vi "ReadNortekFile.vi"(4 "error in":errorcluster, 7 "FichierNortek":path) -> (0 "error out":errorcluster, 2 "Nortek WaveForms":waveform(dbl)[](graph))   [LabVIEW 2017]
uses:
  <vilib>/gmath/NI_Gmath.lvlib
panel:
  out "text":string
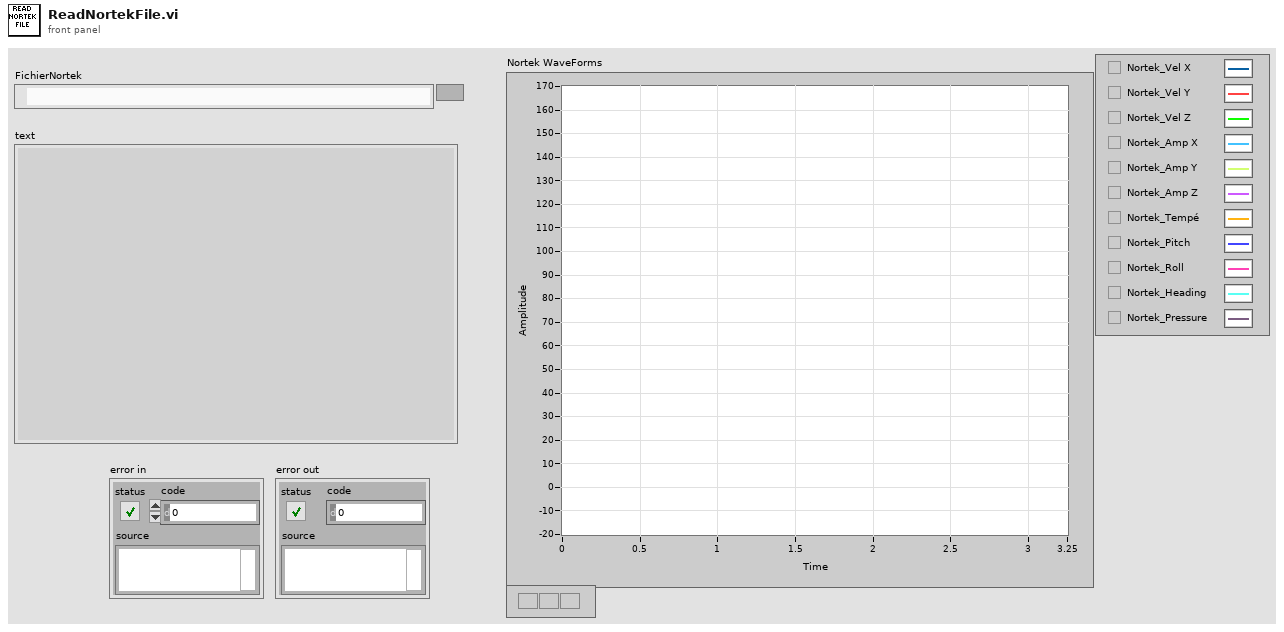
[diagram p1: front panel]
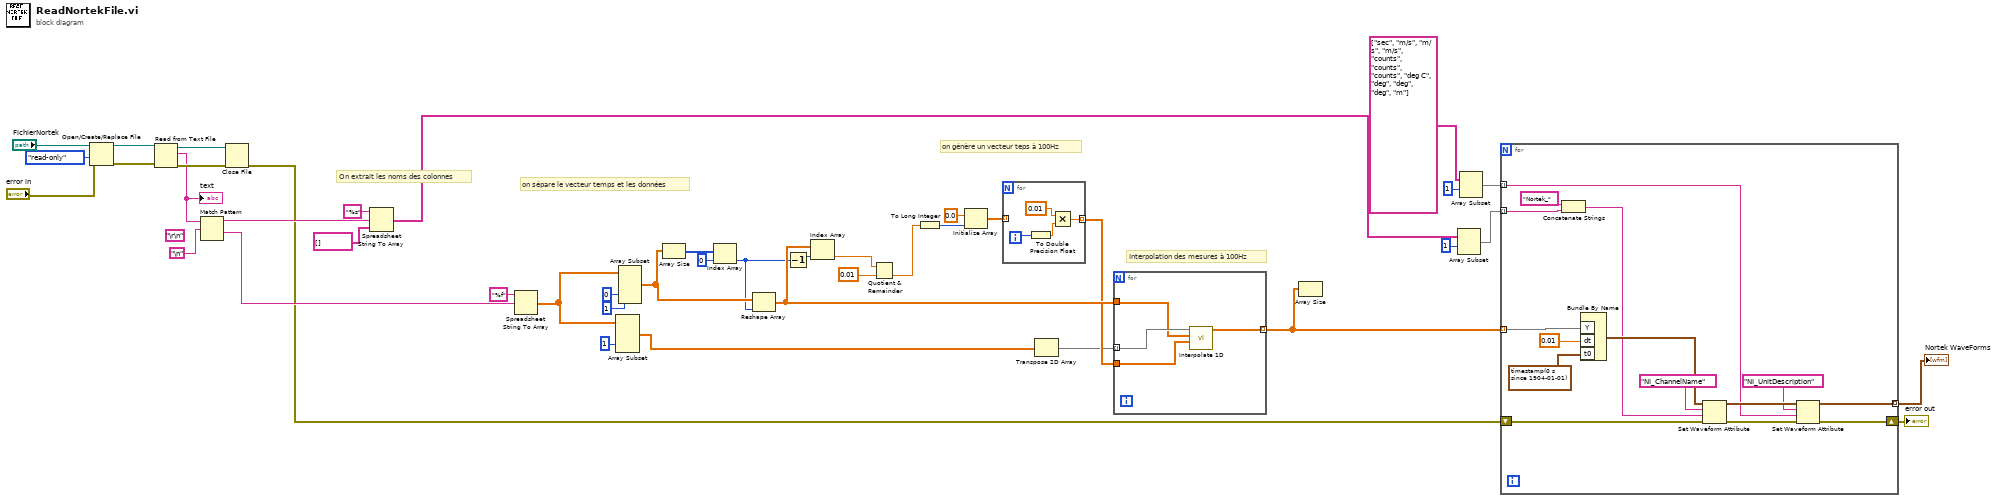
[diagram p0: block diagram]
diagram:
  (unwired) "\r\n"
  # "Interpolation des mesures à 100Hz"
  # "on génère un vecteur teps à 100Hz"
  # "on sépare le vecteur temps et les données"
  # "On extrait les noms des colonnes"
  n1 = Open/Create/Replace File(file path (use dialog)="FichierNortek", error in="error in", access (0:read/write)=enum16{"read/write", "read-only", "write-only"}."read-only") -> (refnum out=w41:refnum<file>, error out=w43:errorcluster)  [unwired: 3 in, 1 out]
  n2 = Read from Text File(file (use dialog)=w41, error in=w43) -> (refnum out=w40:refnum<file>, text=w36:string, error out=w42:errorcluster)  [unwired: 2 in, 1 out]
  "text" <- w36
  n3 = Match Pattern(string=w36, regular expression="\n") -> (before substring=w34:string, after substring=w31:string)  [unwired: 1 in, 2 out]
  n4 = Close File(refnum=w40, error in=w42) -> (error out=w9:errorcluster)  [unwired: 1 out]
  n5 = Spreadsheet String To Array(format string="%s", spreadsheet string=w34, array type (2D Dbl)=string[] []) -> (array=w2:string[])  [unwired: 1 in]
  n6 = Spreadsheet String To Array(format string="%f", spreadsheet string=w31) -> (array=w26:dbl[][])  [unwired: 2 in]
  n7 = Array Subset(array=w26, index (col)=1 ("index")) -> (w25:dbl[][])  [unwired: 3 in]
  n8 = Array Subset(array=w26, index (col)=0 ("index"), length (col)=1 ("length")) -> (w24:dbl[][])  [unwired: 2 in]
  n9 = Array Size(array=w24) -> (size(s)=w23:i32[])
  n10 = Index Array(array=w23, index=0) -> (element=w20:i32)
  n11 = Reshape Array(w24, w20) -> (w21:dbl[])
  n12 = Decrement(x=w20) -> (x-1=w19:i32)
  n13 = Index Array(array=w21, index=w19) -> (element=w18:dbl)
  n14 = Quotient & Remainder(x=w18, y=0.01) -> (floor(x/y)=w16:dbl)  [unwired: 1 out]
  n15 = To Long Integer(number=w16) -> (32bit integer=w15:i32)
  n16 = Initialize Array(0.0 ("element"), w15) -> (w13:dbl[])
  n17 = for {
    tunnel: w13 -> [_] mode=indexing
    tunnel: [w45] -> w12 mode=indexing
    i -> [w46]
    n18 = To Double Precision Float(number=w46) -> (double precision float=w44:dbl)
    n19 = Multiply(x=0.01 ("y"), y=w44) -> (x*y=w45:dbl)
  }
  n20 = Transpose 2D Array(2D array=w25) -> (transposed array=w11:dbl[][])
  n21 = for {
    tunnel: w11 -> [w51] mode=indexing
    tunnel: w21 -> [w50]
    tunnel: w12 -> [w49]
    tunnel: [w48] -> w10 mode=indexing
    n22 = call <vilib>:"Interpolate 1D.vi"("xi"=w49, "X"=w50, "Y"=w51) -> ("yi"=w48:dbl[])  [unwired: 6 in, 2 out]
  }
  n23 = Array Size(array=w10) -> ()  [unwired: 1 out]
  n24 = Array Subset(array=w2, index=1) -> (w1:string[])  [unwired: 1 in]
  n25 = Array Subset(array=string[] ["sec", "m/s", "m/s", "m/s", "counts", "counts", "counts", "deg C", "deg", "deg", "deg", "m"] ("unités"), index=1) -> (w5:string[])  [unwired: 1 in]
  n26 = for {
    tunnel: w10 -> [w64] mode=indexing
    tunnel: w1 -> [w54] mode=indexing
    tunnel: w5 -> [w52] mode=indexing
    shift-right: [w57] -> w7
    shift-left: w9 -> [w59]
    tunnel: [w56] -> w8 mode=indexing
    n27 = Concatenate Strings("Nortek_" ("string"), w54) -> (w53:string)
    n28 = Bundle By Name("Y"=w64, "dt"=0.01, "t0"=timestamp(0 s since 1904-01-01)) -> (w58:waveform(dbl))  [unwired: 1 in]
    n29 = Set Waveform Attribute(4:w59, 5:w53, 6:"NI_ChannelName" ("nom"), 7:w58) -> (0:w62:errorcluster, 3:w63:waveform(dbl))  [unwired: 1 out]
    n30 = Set Waveform Attribute(4:w62, 5:w52, 6:"NI_UnitDescription" ("nom"), 7:w63) -> (0:w57:errorcluster, 3:w56:waveform(dbl))  [unwired: 1 out]
  }
  "Nortek WaveForms" <- w8
  "error out" <- w7
